vi "number2sine-signal.vi"(1 "sample rate\n(44100 sample/s)":dbl=44100.0 format="%#_13g", 2 "index(0~31)":i32, 3 "period(s)":dbl=0.1) -> (0 "signal out":waveform(dbl))   [LabVIEW 2014]
uses:
  <vilib>/measure/NI_MABase.lvlib
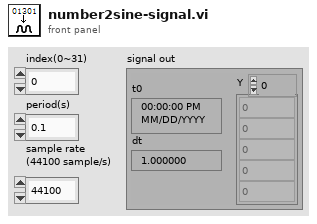
[diagram p1: front panel]
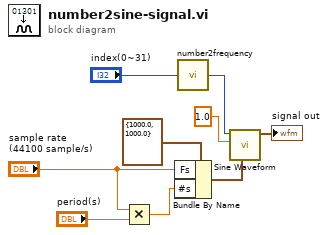
[diagram p0: block diagram]
diagram:
  n1 = Multiply(x="sample rate\n(44100 sample/s)", y="period(s)") -> (x*y=w6:dbl)
  n2 = Bundle By Name(cluster=cluster{"Fs":dbl, "#s":dbl} {"Fs"=1000.0, "#s"=1000.0} ("sampling info"), "Fs"="sample rate\n(44100 sample/s)", "#s"=w6) -> (w4:cluster{"Fs":dbl, "#s":dbl})
  n3 = call "number2frequency.vi"("index(0~31)"="index(0~31)") -> ("Numeric"=w2:i32)
  n4 = call <vilib>:"Sine Waveform.vi"("sampling info"=w4, "amplitude"=1.0, "frequency"=w2) -> ("signal out"=→"signal out":waveform(dbl))  [unwired: 7 in, 1 out]
